vi "Inputs.vi"(8 "error in (no error)":errorcluster, 11 "State in":T1={"State"=enum."Idle", "Start Time"=timestamp(0 s since 1904-01-01), "Configuration"={"Cycle Period"=0.0, "Ismatech"={"VISA resource name"="", "Simulated?"=FALSE, "Pump Number"=1.0, "Reverse?"=FALSE}, "Masterflex"={"VISA resource name"="", "Simulated?"=FALSE, "Pump Number"=1.0, "Reverse?"=FALSE}, "Manual Entry"=0.0, "VICI Settings"={"VISA resource name"="", "Simulated?"=FALSE, "Pump Number"=0.0, "Reverse?"=FALSE}, "Output Device"=enum."Ismatec ISM 831C"}, "Current Time"=timestamp(0 s since 1904-01-01), "First Iteration"=FALSE, "Data"={"Pump Speed"=0.0}, "Process Name"="", "Pump On?"=FALSE} {"Configuration"."VICI Settings"."Pump Number" min=1.0 max=20.0 step=1.0; "Configuration"."Masterflex"."Pump Number" min=1.0 max=20.0 step=1.0; "Configuration"."Ismatech"."Pump Number" min=1.0 max=20.0 step=1.0}) -> (0 "error out":errorcluster, 3 "State out":T1={"State"=enum."Idle", "Start Time"=timestamp(0 s since 1904-01-01), "Configuration"={"Cycle Period"=0.0, "Ismatech"={"VISA resource name"="", "Simulated?"=FALSE, "Pump Number"=1.0, "Reverse?"=FALSE}, "Masterflex"={"VISA resource name"="", "Simulated?"=FALSE, "Pump Number"=1.0, "Reverse?"=FALSE}, "Manual Entry"=0.0, "VICI Settings"={"VISA resource name"="", "Simulated?"=FALSE, "Pump Number"=0.0, "Reverse?"=FALSE}, "Output Device"=enum."Ismatec ISM 831C"}, "Current Time"=timestamp(0 s since 1904-01-01), "First Iteration"=FALSE, "Data"={"Pump Speed"=0.0}, "Process Name"="", "Pump On?"=FALSE} {"Configuration"."VICI Settings"."Pump Number" min=1.0 max=20.0 step=1.0; "Configuration"."Masterflex"."Pump Number" min=1.0 max=20.0 step=1.0; "Configuration"."Ismatech"."Pump Number" min=1.0 max=20.0 step=1.0})   [LabVIEW 2021, in "Pump Module.lvlib" / "Pump Module Engine.lvlib"]
uses:
  Pump Module Engine.lvlib
  Mettler Toledo/Mettler Toledo.lvlib
  Bronkhorst M13 Flow Meter/Bronkhorst M13 Flow Meter.lvlib
  Tag VIs/Tag FGV Operation Enum.ctl
  Shared Variables/Dynamic Shared Variables.lvlib
  State Enum.ctl
  Pump Module Settings Cluster.ctl
  Pump Module.lvlib
  State Cluster.ctl
  Measure Instrument/PID 2 Output Enum.ctl
  Ismatec ISM 831C/Controls/Ismatech Settings Cluster.ctl
  Masterflex 7550-30/Controls/Settings Cluster.ctl
  Masterflex 7550-30/Masterflex 7550-30.lvlib
  VICI M50/VICI Settings.ctl
panel:
  # "Output Instruments"
  # "Output Instruments"
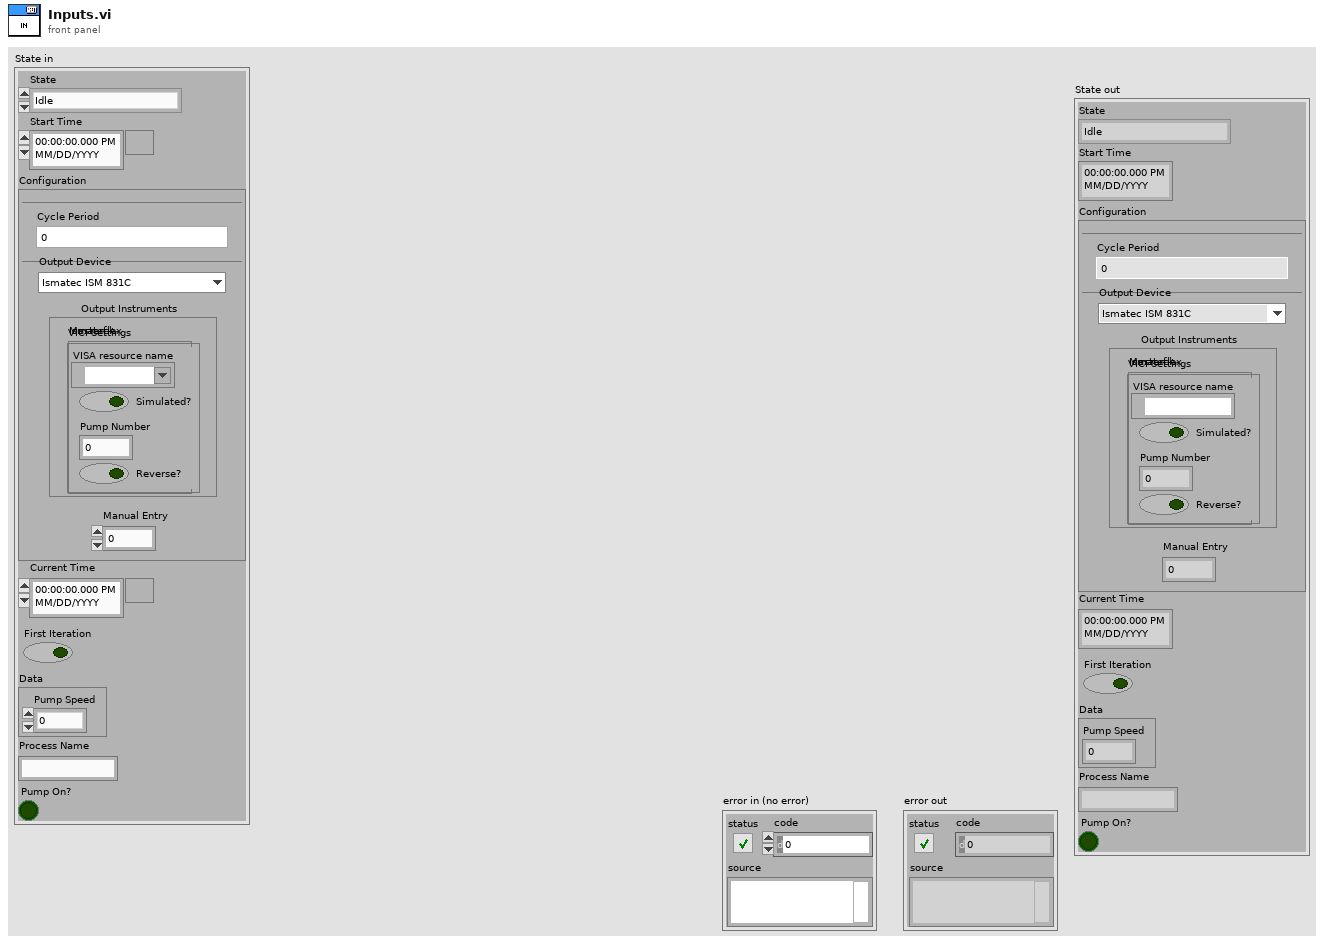
[diagram p1: front panel]
types:
  T1 = typedef "Pump Module.lvlib/Pump Module Engine.lvlib/State Cluster.ctl" = cluster{"State":T2, "Start Time":timestamp, "Configuration":T3, "Current Time":timestamp, "First Iteration":bool, "Data":cluster{"Pump Speed":dbl}, "Process Name":string, "Pump On?":bool}
  T2 = typedef "Pump Module.lvlib/Pump Module Engine.lvlib/State Enum.ctl" = enum16{"Measuring", "Idle", "Paused"}
  T3 = typedef "Pump Module.lvlib/Pump Module Settings Cluster.ctl" = cluster{"Cycle Period":dbl, "Ismatech":T4, "Masterflex":T5, "Manual Entry":dbl, "VICI Settings":T6, "Output Device":T7}
  T4 = typedef "Ismatec ISM 831C.lvlib/Ismatech Settings Cluster.ctl" = cluster{"VISA resource name":refnum<visa-resource-name>, "Simulated?":bool, "Pump Number":dbl, "Reverse?":bool}
  T5 = typedef "Masterflex 7550-30.lvlib/Settings Cluster.ctl" = cluster{"VISA resource name":refnum<visa-resource-name>, "Simulated?":bool, "Pump Number":dbl, "Reverse?":bool}
  T6 = typedef "VICI Settings.ctl" = cluster{"VISA resource name":refnum<visa-resource-name>, "Simulated?":bool, "Pump Number":dbl, "Reverse?":bool}
  T7 = typedef "PID 2 Output Enum.ctl" = enum16{"Default", "Ismatec ISM 4308", "Ismatec ISM 831C", "Masterflex 7550-30", "VICI M6", "VICI M50", "Tacmina QI", "KNF SIMDOS", "ASIA Type C", "FLOM UI-22-11", "SSI PR/LD", "SSI P40", "Masterflex 75211-70"}
  T8 = typedef "Tag FGV Operation Enum.ctl" = enum16{"Init", "Set Notification Queue", "Create Tag", "Commit", "Write Tag (Numeric)", "Write Tag (Boolean)", "Read All Tags", "Read One Tag", "Delete Tag Category", "Set Alarm Parameters (Numeric)", "Set Alarm Parameters (Boolean)", "Enable All Alarms", "Disable All Alarms", "Delete All Tags", "Read Alarms", "Ack Alarm", "Read Alarm Parameters (Numeric)", "Read Alarm Parameters (Boolean)"}
  T9 = typedef "PID Input Enum.ctl" = enum16{"Default", "Flowmeter", "Scale Rate of Change"}
  T10 = typedef "Mettler Toledo.lvlib/Settings Cluster.ctl" = cluster{"VISA resource name":refnum<visa-resource-name>, "Simulated?":bool}
  T11 = typedef "Bronkhorst M13 Flow Meter.lvlib/Settings Cluster.ctl" = cluster{"VISA resource name":refnum<visa-resource-name>, "Simulated?":bool}
  T12 = typedef "Bronkhorst M13 Flow Meter.lvlib/Settings Cluster.ctl" = cluster{"VISA resource name":refnum<visa-resource-name>, "Simulated?":bool, "Smoothing Steps":i32}
  T13 = typedef "Pump Module.lvlib/Pump Module Tag Names Cluster.ctl" = cluster{"Pump Speed":string, "Totalized g Tag":string, "Pump Flow":string, "Pump Pressure":string, "Output Device Tag":string, "Overpressure Tag":string, "Identifier Tag":string}
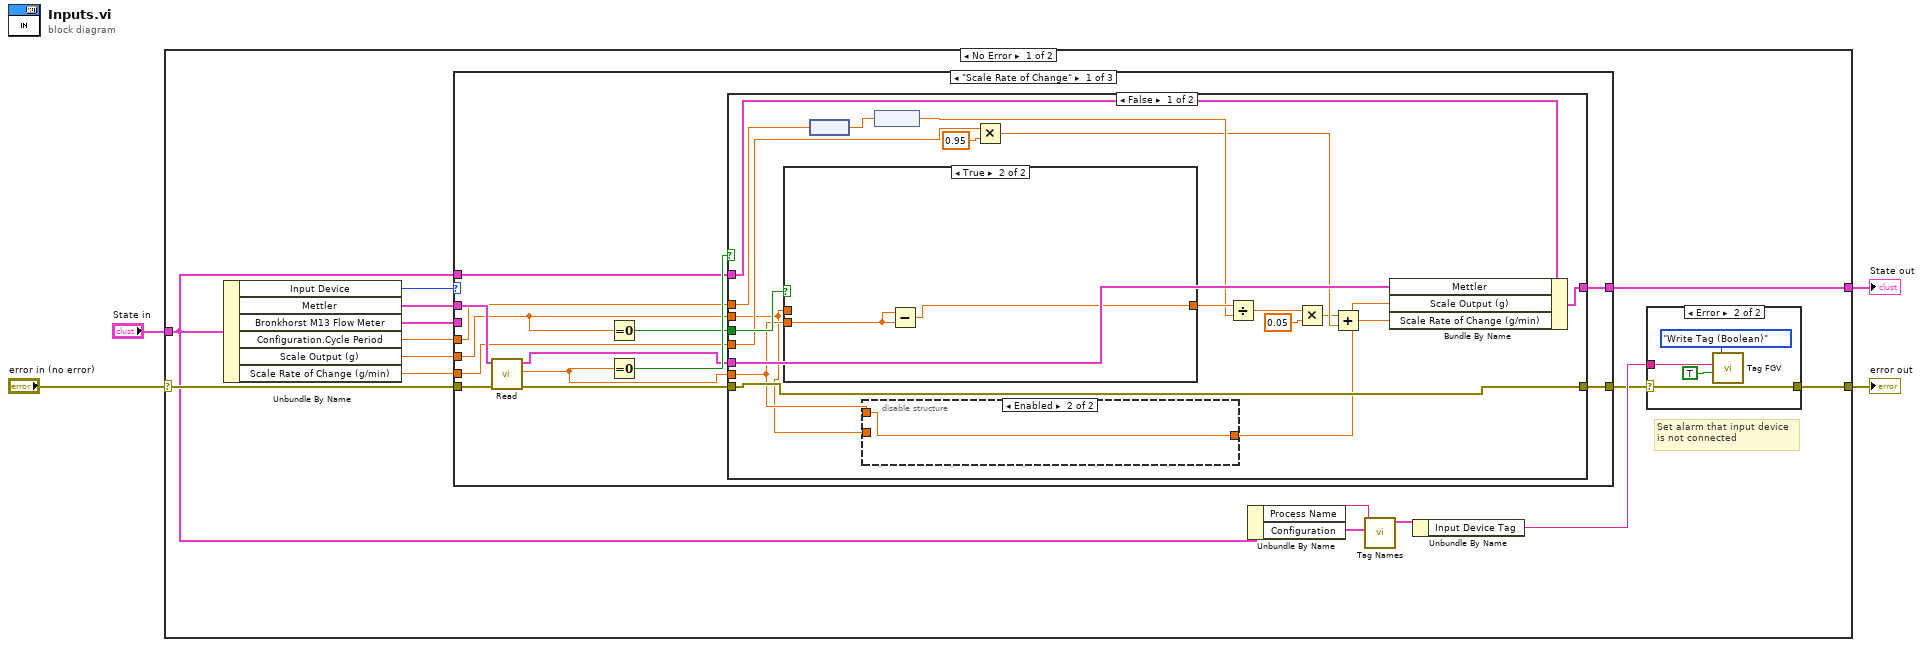
[diagram p0: block diagram]
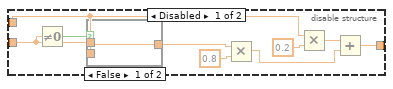
[diagram p3: hidden frame]
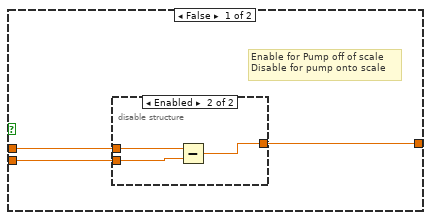
[diagram p5: hidden frame]
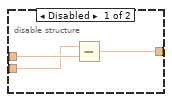
[diagram p6: hidden frame]
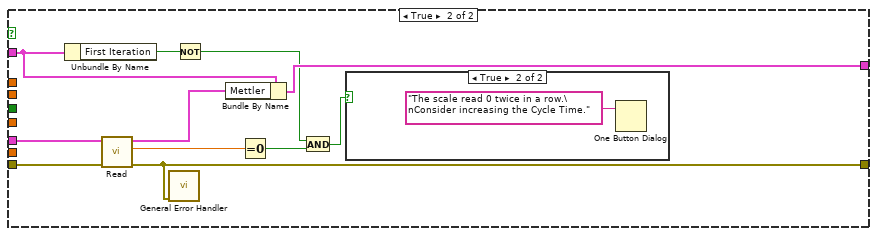
[diagram p7: hidden frame]
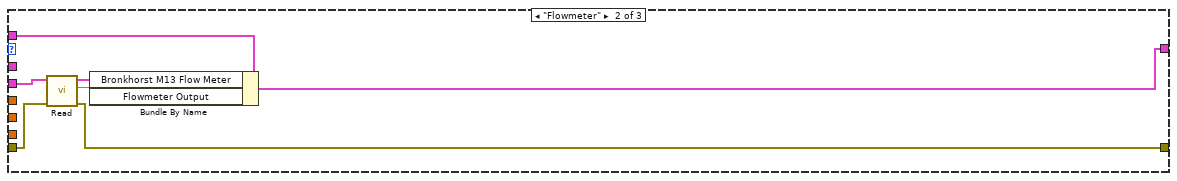
[diagram p9: hidden frame]
diagram:
  n1 = case shown="No Error" "error in (no error)" {
    selector: "error in (no error)" -> [w14 w102]
    tunnel: [w5 w102] -> w1
    tunnel: "State in" -> [w8 w101]
    tunnel: [w18 w101] -> w2
    frame No Error {
      # "Set alarm that input device\nis not connected"
      n2 = Unbundle By Name(w8) -> ("Input Device"=w19:T9, "Mettler"=w17:T10, "Bronkhorst M13 Flow Meter"=w16:T11, "Configuration.Cycle Period"=w15:dbl, "Scale Output (g)"=w13:dbl, "Scale Rate of Change (g/min)"=w12:dbl)
      n3 = case shown="\"Scale Rate of Change\"" w19 {
        tunnel: w8 -> [w32 w98 w100]
        tunnel: [w28 w97 w100] -> w18
        tunnel: w17 -> [w36 _ _]
        tunnel: w16 -> [_ w92 _]
        tunnel: w15 -> [w29 _ _]
        tunnel: w14 -> [w37 w95 w99]
        tunnel: [w26 w94 w99] -> w6
        tunnel: w13 -> [w30 _ _]
        tunnel: w12 -> [w25 _ _]
        frame "Scale Rate of Change" {
          n4 = call "Read.vi"("error in (no error)"=w37, "Mettler Settings in"=w36) -> ("error out"=w27:errorcluster, "mass (g)"=w31:dbl, "Mettler Settings out"=w33:T10)  [unwired: 6 in, 1 out]
          n5 = Equal To 0?(x=w30) -> (x = 0?=w34:bool)
          n6 = Equal To 0?(x=w31) -> (x = 0?=w35:bool)
          n7 = case shown="False" w35 {
            tunnel: w31 -> [w39 _]
            tunnel: w30 -> [w38 _]
            tunnel: w32 -> [w56 w85]
            tunnel: w33 -> [w55 w89]
            tunnel: [w54 w90] -> w28
            tunnel: w29 -> [w51 _]
            tunnel: w34 -> [w49 _]
            tunnel: w27 -> [w48 w87]
            tunnel: [w48 w80] -> w26
            tunnel: w25 -> [w40 _]
            frame False {
              n8 = case shown="True" w49 {
                tunnel: [w70 w79] -> w53
                tunnel: w39 -> [w69 w78]
                tunnel: w38 -> [w71 _]
                frame False {
                  # "Enable for Pump off of scale\nDisable for pump onto scale"
                  n9 = disable-structure shown="Enabled" {
                    disable-tunnel: w71 -> [w74 w76]
                    disable-tunnel: w69 -> [w73 w77]
                    disable-tunnel: [w72 w75] -> w70
                    frame Disabled {
                      n10 = Subtract(x=w73, y=w74) -> (x-y=w72:dbl)
                    }
                    frame Enabled {
                      n11 = Subtract(x=w76, y=w77) -> (x-y=w75:dbl)
                    }
                  }
                }
                frame True {
                  n12 = Subtract(x=w78, y=w78) -> (x-y=w79:dbl)
                }
              }
              n13 = node(w51) -> (w50:dbl[unit])
              n14 = disable-structure shown="Enabled" {
                disable-tunnel: [w61 w68] -> w41
                disable-tunnel: w39 -> [w58 w68]
                disable-tunnel: w38 -> [w57 _]
                frame Disabled {
                  n15 = Not Equal To 0?(x=w57) -> (x != 0?=w59:bool)
                  n16 = case shown="False" w59 {
                    tunnel: w57 -> [_ w67]
                    tunnel: [w66 w67] -> w60
                    tunnel: w58 -> [w66 _]
                    frame False {
                    }
                    frame True {
                    }
                  }
                  n17 = Multiply(x=w60, y=0.8) -> (x*y=w62:dbl)
                  n18 = Multiply(x=w58, y=0.2) -> (x*y=w63:dbl)
                  n19 = Add(x=w63, y=w62) -> (x+y=w61:dbl)
                }
                frame Enabled {
                }
              }
              n20 = node(w50) -> (w52:dbl)
              n21 = Multiply(x=w40, y=0.95) -> (x*y=w47:dbl)
              n22 = Divide(x=w53, y=w52) -> (x/y=w43:dbl)
              n23 = Multiply(x=w43, y=0.05) -> (x*y=w44:dbl)
              n24 = Add(x=w44, y=w47) -> (x+y=w42:dbl)
              n25 = Bundle By Name(cluster=w56, "Mettler"=w55, "Scale Output (g)"=w41, "Scale Rate of Change (g/min)"=w42) -> (w54:T1)
            }
            frame True {
              n26 = Unbundle By Name(w85) -> ("First Iteration"=w84:bool)
              n27 = call "Read.vi"("error in (no error)"=w87, "Mettler Settings in"=w89) -> ("error out"=w80:errorcluster, "mass (g)"=w86:dbl, "Mettler Settings out"=w88:T10)  [unwired: 6 in, 1 out]
              n28 = call <vilib>:"General Error Handler.vi"("error in (no error)"=w80) -> ()  [unwired: 10 in, 5 out]
              n29 = Not(x=w84) -> (.not. x?=w83:bool)
              n30 = Bundle By Name(cluster=w85, "Mettler"=w88) -> (w90:T1)
              n31 = Equal To 0?(x=w86) -> (x = 0?=w82:bool)
              n32 = And(x=w83, y=w82) -> (x .and. y?=w81:bool)
              n33 = case shown="True" w81 {
                frame False {
                }
                frame True {
                  n34 = One Button Dialog(message="The scale read 0 twice in a row.\nConsider increasing the Cycle Time.") -> ()  [unwired: 1 in, 1 out]
                }
              }
            }
          }
        }
        frame "Flowmeter" {
          n35 = call "Read.vi"("error in (no error)"=w95, "Bronkhorst Settings in"=w92) -> ("error out"=w94:errorcluster, "flow"=w96:dbl, "Bronkhorst Settings out"=w93:T12)  [unwired: 6 in, 1 out]
          n36 = Bundle By Name(cluster=w98, "Bronkhorst M13 Flow Meter"=w93, "Flowmeter Output"=w96) -> (w97:T1)
        }
        frame "Default", Default {
        }
      }
      n37 = Unbundle By Name(w8) -> ("Process Name"=w10:string, "Configuration"=w11:T3)
      n38 = call "Tag Names.vi"(10:w11, "State In"=w10) -> ("Pump Module Tag Names"=w9:T13)  [unwired: 7 in, 2 out]
      n39 = Unbundle By Name(w9) -> ("Input Device Tag"=w7:string)
      n40 = case shown="Error" w6 {
        selector: w6 -> [w20 w22]
        tunnel: [w20 w22] -> w5
        tunnel: w7 -> [_ w21]
        frame No Error {
        }
        frame Error {
          n41 = call "Tag FGV.vi"("Data"=TRUE, "Tag Name"=w21, "Operation"=Tag_FGV_Operation_Enum."Write Tag (Boolean)") -> ()  [unwired: 3 in, 6 out]
        }
      }
    }
    frame Error {
    }
  }
  "error out" <- w1
  "State out" <- w2
